vi "RawTrace.vi"() -> ()   [LabVIEW 2021, in "YActor.lvclass"]
uses:
  YActor.lvclass
  tracing/TraceDefinition.ctl
panel:
  in  "TraceEnable":T1
  in  "RawTrace":refnum<file>
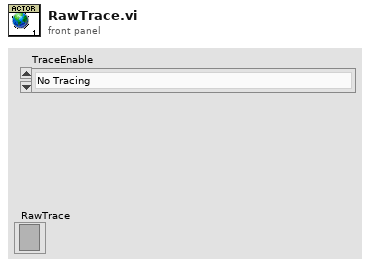
[diagram p1: front panel]
types:
  T1 = typedef "YActor.lvclass/TraceDefinition.ctl" = enum16{"No Tracing", "Basic", "Basic + Method IO", "Basic + Method IO + Object in", "Basic + Method IO + Object IO"}
diagram:
